vi "DFD FXP Quantize Coef (Advanced).vi"(5 "coefficients b/v quantizer":T2={"source"=7, "wl"=-1, "iwl"=1, "overflow mode"=enum."Saturation", "rounding mode"=enum."Nearest", "signed?"=TRUE} {"source" items=["Coefficients a/k"=0, "Coefficients b/v"=7, "Input"=1, "Output"=2, "Multiplicand"=3, "Product"=4, "Sum"=5, "Delay"=6]}, 6 "gain settings":T1={"gain processing"=1, "gain word length"=16} {"gain processing" items=["On Target", "On Host"]}, 7 "coefficients a/k quantizer":T2={"source"=0, "wl"=16, "iwl"=1, "overflow mode"=enum."Saturation", "rounding mode"=enum."Nearest", "signed?"=TRUE} {"source" items=["Coefficients a/k"=0, "Coefficients b/v"=7, "Input"=1, "Output"=2, "Multiplicand"=3, "Product"=4, "Sum"=5, "Delay"=6]}, 8 "error in (no error)":errorcluster, 11 "filter in":T4={"mSRate_Fs"=1.0, "mSRate_Version"="2.0", "mSRate_Comments"="", "mSRate_OrgCoef"={"type"=enum."Undefined", "gain"=1.0, "coef a (k)"=[], "coef b (v)"=[]}, "mSRate_CurCoef"={"type"=enum."Undefined", "gain"=1.0, "coef a (k)"=[], "coef b (v)"=[]}, "mSRate_Quantized?"=FALSE, "mSRate_QCoef"={"type"=enum."Undefined", "gain"=1.0, "coef a (k)"=[], "coef b (v)"=[]}, "mSRate_QSettings"=[], "mSRate_Order"=0, "mSRate_Scaling"={"mSRate_ScaleByPowerOf2?"=FALSE, "mSRate_ScaleType"=enum."No Norm"}} {"mSRate_QSettings"."source" items=["Coef a/k"=0, "Coef b/v"=7, "Input"=1, "Output"=2, "Multiplicand"=3, "Product"=4, "Sum"=5, "Delay"=6, "Gain"=8]}) -> (0 "error out":errorcluster, 3 "filter out":T4={"mSRate_Fs"=1.0, "mSRate_Version"="2.0", "mSRate_Comments"="", "mSRate_OrgCoef"={"type"=enum."Undefined", "gain"=1.0, "coef a (k)"=[], "coef b (v)"=[]}, "mSRate_CurCoef"={"type"=enum."Undefined", "gain"=1.0, "coef a (k)"=[], "coef b (v)"=[]}, "mSRate_Quantized?"=FALSE, "mSRate_QCoef"={"type"=enum."Undefined", "gain"=1.0, "coef a (k)"=[], "coef b (v)"=[]}, "mSRate_QSettings"=[], "mSRate_Order"=0, "mSRate_Scaling"={"mSRate_ScaleByPowerOf2?"=FALSE, "mSRate_ScaleType"=enum."No Norm"}} {"mSRate_QSettings"."source" items=["Coef a/k"=0, "Coef b/v"=7, "Input"=1, "Output"=2, "Multiplicand"=3, "Product"=4, "Sum"=5, "Delay"=6, "Gain"=8]})   [LabVIEW 2017, in "NI_DigFilterLicensed.lvlib"]
doc: "Quantizes the coefficients of a floating-point filter and generates a fixed-point filter. You must manually select the polymorphic instance you want to use."
uses:
  <vilib>/addons/Digital Filter Design/NI_DigFilterLicensed.lvlib
  <vilib>/addons/Digital Filter Design/_Objects.llb/DFD Filter Obj.ctl
  <vilib>/addons/Digital Filter Design/_Objects.llb/DFD Filter Coef.ctl
  <vilib>/addons/Digital Filter Design/_Objects.llb/DFD Filter Structure Type Selector.ctl
  <vilib>/addons/Digital Filter Design/_Objects.llb/dfd_Internal Quantization Settings.ctl
  <vilib>/addons/Digital Filter Design/_Objects.llb/dfd_Internal Quantization Srcs.ctl
  <vilib>/addons/Digital Filter Design/_Objects.llb/DFD Coef Norm Type.ctl
  <vilib>/addons/Digital Filter Design/_Objects.llb/DFD Quantization Settings.ctl
  <vilib>/addons/Digital Filter Design/_Objects.llb/DFD Quantization Sources.ctl
  <vilib>/addons/Digital Filter Design/_Objects.llb/DFD Round-off Mode.ctl
  <vilib>/addons/Digital Filter Design/NI_DigFilter_FXP.lvlib
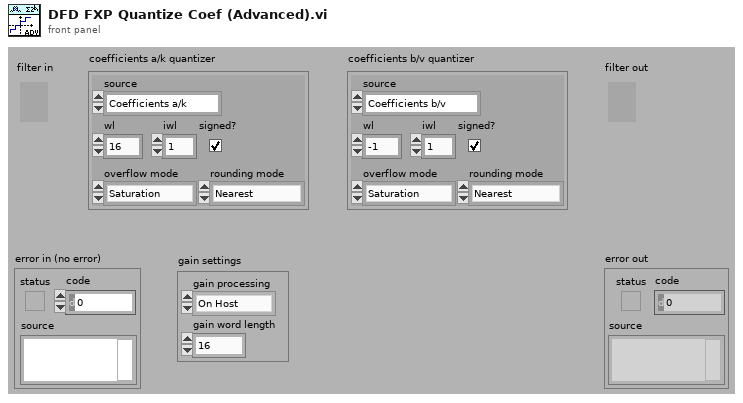
[diagram p1: front panel]
types:
  T1 = cluster{"gain processing":u16, "gain word length":i16}
  T2 = typedef "NI_DigFilterLicensed.lvlib/DFD Quantization Settings.ctl" = cluster{"source":T3, "wl":i16, "iwl":i16, "overflow mode":enum16{"Saturation", "Wrap"}, "rounding mode":enum16{"Nearest", "Truncation"}, "signed?":bool}
  T3 = typedef "NI_DigFilterLicensed.lvlib/DFD Quantization Sources.ctl" = u16
  T4 = typedef "NI_DigFilterLicensed.lvlib/DFD Filter Obj.ctl" = cluster{"mSRate_Fs":dbl, "mSRate_Version":string, "mSRate_Comments":string, "mSRate_OrgCoef":T5, "mSRate_CurCoef":T5, "mSRate_Quantized?":bool, "mSRate_QCoef":T5, "mSRate_QSettings":T7[], "mSRate_Order":i32, "mSRate_Scaling":cluster{"mSRate_ScaleByPowerOf2?":bool, "mSRate_ScaleType":T9}}
  T5 = typedef "NI_DigFilterLicensed.lvlib/DFD Filter Coef.ctl" = cluster{"type":T6, "gain":dbl, "coef a (k)":dbl[], "coef b (v)":dbl[]}
  T6 = typedef "NI_DigFilterLicensed.lvlib/DFD Filter Structure Type Selector.ctl" = enum16{"Undefined", "FIR Direct Form", "FIR Direct Form Transposed", "FIR Symmetric", "FIR Antisymmetric", "IIR Direct Form I", "IIR Direct Form I Transposed", "IIR Direct Form II", "IIR Direct Form II Transposed", "IIR Cascaded Second Order Sections Form I", "IIR Cascaded Second Order Sections Form I Transposed", "IIR Cascaded Second Order Sections Form II", "IIR Cascaded Second Order Sections Form II Transposed", "Lattice Allpass (basic sections)", "Lattice Allpass (one multiplier sections)", "Lattice Allpass (normalized sections)", "Lattice AR (basic sections)", "Lattice AR (one multiplier sections)", "Lattice AR (normalized sections)", "Lattice MA (minimum phase)", "Lattice MA (maximum phase)", "Lattice ARMA (basic sections)", "Lattice ARMA (one multiplier sections)", "Lattice ARMA (normalized sections)"}
  T7 = typedef "NI_DigFilterLicensed.lvlib/dfd_Internal Quantization Settings.ctl" = cluster{"source":T8, "wl":i16, "iwl":i16, "overflow mode":enum16{"Saturation", "Wrap"}, "rounding mode":enum16{"Nearest", "Truncation"}, "signed?":bool}
  T8 = typedef "NI_DigFilterLicensed.lvlib/dfd_Internal Quantization Srcs.ctl" = u16
  T9 = typedef "NI_DigFilterLicensed.lvlib/DFD Coef Norm Type.ctl" = enum16{"No Norm", "Time Domain 1-Norm", "Time Domain 2-Norm", "Time Domain Inf-Norm"}
  T10 = typedef "NI_DigFilterLicensed.lvlib/DFD Round-off Mode.ctl" = enum16{"Nearest", "Truncation"}
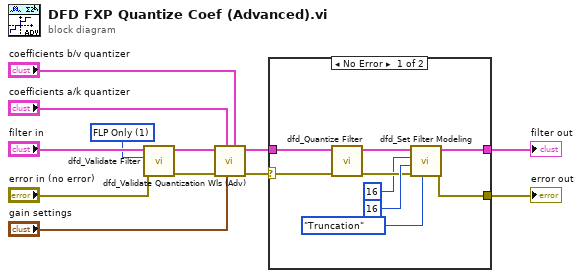
[diagram p0: block diagram]
diagram:
  w2 = u16 1 items=["Auto", "FLP Only", "FXP"] ("check option")
  n1 = call <vilib>:"dfd_Validate Filter.vi"("error in (no error)"="error in (no error)", "check option"=w2, "filter in"="filter in") -> ("error out"=w4:errorcluster, "filter out"=w5:T4)  [unwired: 7 out]
  n2 = call <vilib>:"dfd_Validate Quantization Wls (Adv).vi"("Coef b/v quantizer"="coefficients b/v quantizer", "gain setting"="gain settings", "Coef a/k quantizer"="coefficients a/k quantizer", "error in (no error)"=w4, "filter in"=w5) -> ("error out"=w1:errorcluster, "filter out"=w3:T4)  [unwired: 5 out]
  n3 = case shown="No Error" w1 {
    selector: w1 -> [w13 w22]
    tunnel: [w21 _] -> w12
    tunnel: [w20 w22] -> w7
    tunnel: w3 -> [w19 _]
    frame No Error {
      n4 = call <vilib>:"dfd_Quantize Filter.vi"("error in (no error)"=w13, "filter in"=w19) -> ("error out"=w15:errorcluster, "filter out"=w16:T4)  [unwired: 8 out]
      n5 = call <vilib>:"dfd_Set Filter Modeling.vi"("output round-off mode"=DFD_Round-off_Mode."Truncation", "error in (no error)"=w15, "output wl (16)"=i16 16, "input wl (16)"=i16 16, "filter in"=w16) -> ("error out"=w20:errorcluster, "filter out"=w21:T4)  [unwired: 2 in, 3 out]
    }
    frame Error {
    }
  }
  "filter out" <- w12
  "error out" <- w7
